vi "Measurement Logic.vi"() -> ()   [LabVIEW 2024, in "NIScopeFrequencyDomain.lvlib"]
uses:
  NIScopeFrequencyDomain.lvlib
  Measurement Configuration.ctl
  Measurement Results.ctl
  <vilib>/gRPC/Generated APIs/ni/protobuf/types/RPC Messages/ni_protobuf_types_DoubleXYData.ctl
  <vilib>/MeasurementLink/MeasurementLink Measurement Server/Measure Call Context/Measure Call Context.lvclass
  <vilib>/MeasurementLink/MeasurementLink Measurement Server/Measure Call Context/Reserve Sessions - 1Pin.vi
  <vilib>/MeasurementLink/MeasurementLink niScope/Initialize Sessions - 1Sess.vi
  <vilib>/MeasurementLink/MeasurementLink niScope/Get Connections - 1Pin 1Conn.vi
  <instrlib>/niScope/Configure/Trigger/niScope Configure Trigger Edge.vi
  <instrlib>/niScope/Acquire/Fetch/niScope Fetch WDT.vi
  <vilib>/MeasurementLink/MeasurementLink niScope/MeasurementLink niScope.lvlib
  <vilib>/gRPC/Generated APIs/ni/protobuf/types/ni.protobuf.types.lvlib
  <vilib>/MeasurementLink/MeasurementLink Session Management V1/Session Reservation/Session Reservation.lvclass
panel:
  out "measure call context out":refnum<class "Measure Call Context.lvclass">
  in  "measure call context in":refnum<class "Measure Call Context.lvclass">
  out "measurement results":T1
  in  "measurement configuration":T3={"Pin Name"="", "Vertical Range (V)"=10.0, "Vertical Offset (V)"=0.0, "Vertical Coupling"=1, "Minimum Sample Rate (S/s)"=10000.0, "Minimum Record Length (S)"=20000, "Trigger Level (V)"=0.0, "Trigger Coupling"=1, "Trigger Slope"=0} {"Trigger Slope" items=["Positive", "Negative"]; "Trigger Coupling" items=["AC"=0, "DC"=1, "HF Reject"=3, "LF Reject"=4, "AC Plus HF Reject"=1001]; "Trigger Level (V)" format="%.2g"; "Minimum Sample Rate (S/s)" format="%#.5p"; "Vertical Coupling" items=["AC", "DC", "Ground"]; "Vertical Offset (V)" format="%.2p"; "Vertical Range (V)" format="%.2f"}
  out "error out":errorcluster
  in  "error in":errorcluster
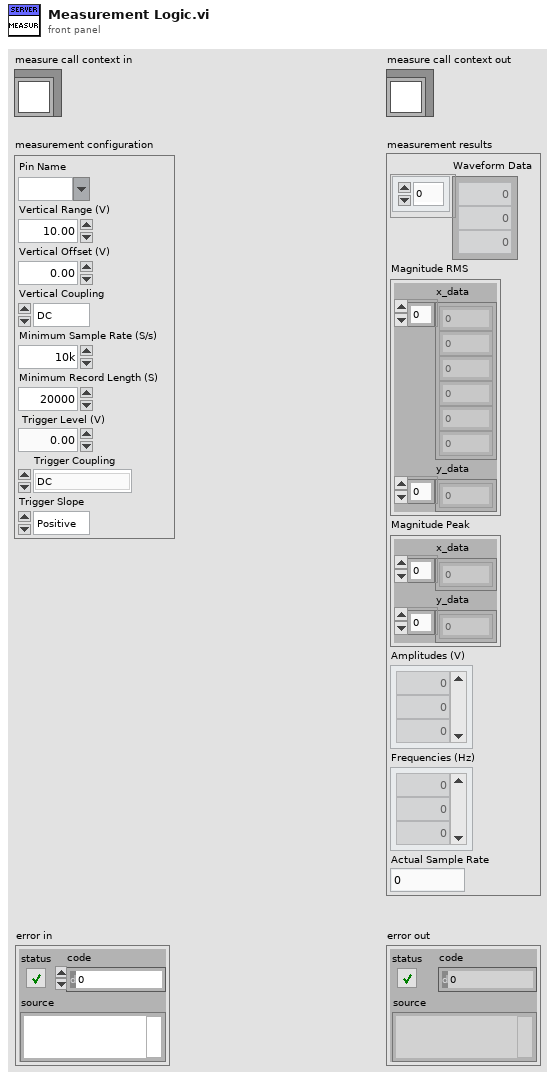
[diagram p1: front panel]
types:
  T1 = typedef "NIScopeFrequencyDomain.lvlib/Measurement Results.ctl" = cluster{"Waveform Data":dbl[], "Magnitude RMS":T2, "Magnitude Peak":T2, "Amplitudes (V)":dbl[], "Frequencies (Hz)":dbl[], "Actual Sample Rate":dbl}
  T2 = typedef "ni.protobuf.types.lvlib/ni_protobuf_types_DoubleXYData.ctl" = cluster{"x_data":dbl[], "y_data":dbl[]}
  T3 = typedef "NIScopeFrequencyDomain.lvlib/Measurement Configuration.ctl" = cluster{"Pin Name":string, "Vertical Range (V)":dbl, "Vertical Offset (V)":dbl, "Vertical Coupling":i32, "Minimum Sample Rate (S/s)":dbl, "Minimum Record Length (S)":i32, "Trigger Level (V)":dbl, "Trigger Coupling":u32, "Trigger Slope":i32}
  T4 = typedef "MeasurementLink niScope.lvlib/Connection with Session.ctl" = cluster{"connection":T5, "session":refnum<k15>}
  T5 = typedef "MeasurementLink Session Management V1.lvlib/Session Reservation.lvclass/Connection.ctl" = cluster{"pin or relay name":string, "site":i32, "instrument type id":string, "channel":string}
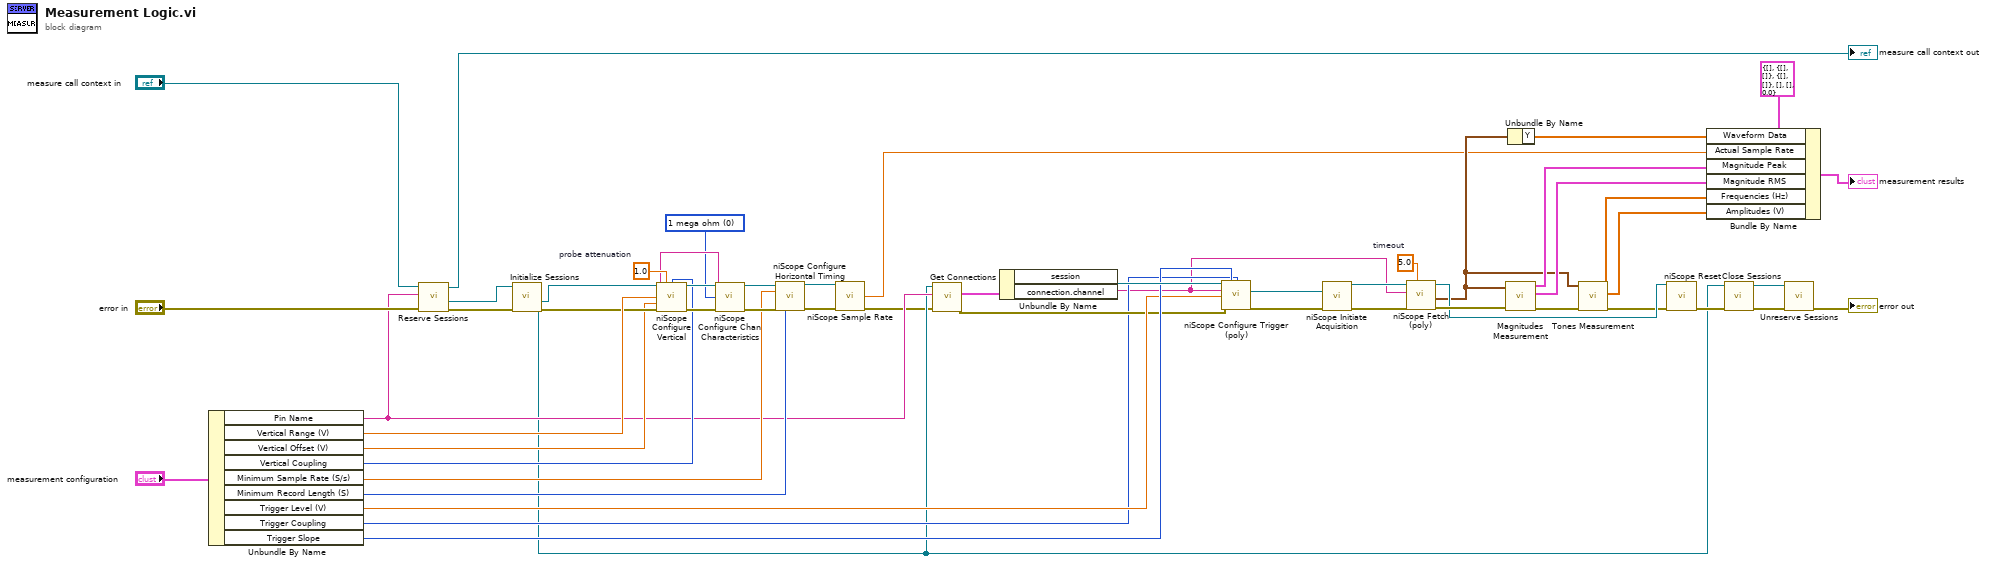
[diagram p0: block diagram]
diagram:
  w13 = u32 0 items=["1 mega ohm"=0, "50 ohms"=2] ("input impedance")
  w24 = 5.0  # timeout
  w44 = 1.0  # probe attenuation
  n1 = Unbundle By Name("measurement configuration") -> ("Pin Name"=w35:string, "Vertical Range (V)"=w47:dbl, "Vertical Offset (V)"=w45:dbl, "Vertical Coupling"=w36:i32, "Minimum Sample Rate (S/s)"=w38:dbl, "Minimum Record Length (S)"=w37:i32, "Trigger Level (V)"=w31:dbl, "Trigger Coupling"=w29:u32, "Trigger Slope"=w32:i32)
  n2 = call-poly <vilib>:"Reserve Sessions.vi"("error in"="error in", "pin or relay name"=w35, "measurement context in"="measure call context in") -> ("error out"=w49:errorcluster, "session reservation out"=w51:refnum<class "Session Reservation.lvclass">, "measurement context out"=→"measure call context out":refnum<class "Measure Call Context.lvclass">)  [unwired: 6 in]
  n3 = call-poly <vilib>:"Initialize Sessions.vi"("error in"=w49, "session reservation in"=w51) -> ("error out"=w46:errorcluster, "channel list"=w41:string, "session"=w48:refnum<k15>, "session reservation out"=w17:refnum<class "Session Reservation.lvclass">)  [unwired: 6 in]
  n4 = call <instrlib>:"niScope Configure Vertical.vi"("instrument handle"=w48, "probe attenuation"=w44, "vertical coupling"=w36, "channels"=w41, "vertical range"=w47, "vertical offset"=w45, "error in"=w46) -> ("instrument handle out"=w43:refnum<k15>, "error out"=w42:errorcluster)  [unwired: 7 in]
  n5 = call <instrlib>:"niScope Configure Chan Characteristics.vi"("instrument handle"=w43, "channels"=w41, "input impedance"=w13, "error in"=w42) -> ("instrument handle out"=w40:refnum<k15>, "error out"=w39:errorcluster)  [unwired: 10 in]
  n6 = call <instrlib>:"niScope Configure Horizontal Timing.vi"("instrument handle"=w40, "min sample rate"=w38, "error in"=w39, "min record length"=w37) -> ("instrument handle out"=w5:refnum<k15>, "error out"=w4:errorcluster)  [unwired: 10 in]
  n7 = call <instrlib>:"niScope Sample Rate.vi"("instrument handle"=w5, "error in"=w4) -> ("actual sample rate"=w1:dbl, "error out"=w3:errorcluster)  [unwired: 11 in, 1 out]
  n8 = call-poly <vilib>:"Get Connections.vi"("error in"=w3, "pin or relay name"=w35, "session reservation in"=w17) -> ("error out"=w30:errorcluster, "connection"=w34:T4)  [unwired: 6 in, 1 out]
  n9 = Unbundle By Name(w34) -> ("session"=w33:refnum<k15>, "connection.channel"=w23:string)
  n10 = call-poly <instrlib>:"niScope Configure Trigger (poly).vi"("instrument handle"=w33, "trigger slope"=w32, "trigger coupling"=w29, "trigger source"=w23, "trigger level"=w31, "error in"=w30) -> ("instrument handle out"=w28:refnum<k15>, "error out"=w27:errorcluster)  [unwired: 8 in]
  n11 = call <instrlib>:"niScope Initiate Acquisition.vi"("instrument handle"=w28, "error in"=w27) -> ("instrument handle out"=w26:refnum<k15>, "error out"=w25:errorcluster)  [unwired: 12 in]
  n12 = call-poly <instrlib>:"niScope Fetch (poly).vi"("timeout"=w24, "error in"=w25, "channels"=w23, "instrument handle"=w26) -> ("error out"=w20:errorcluster, "wfm"=w10:waveform(dbl), "instrument handle out"=w19:refnum<k15>)  [unwired: 4 in, 1 out]
  n13 = call "Magnitudes Measurement.vi"("error in"=w20, "wfm"=w10) -> ("error out"=w9:errorcluster, "Magnitude RMS"=w11:cluster{dbl[], "magnitude":dbl[]}, "Magnitude Peak"=w12:cluster{dbl[], dbl[]})  [unwired: 7 in]
  n14 = Unbundle By Name(w10) -> ("Y"=w2:dbl[])
  n15 = call "Tones Measurement.vi"("error in"=w9, "wfm"=w10) -> ("error out"=w8:errorcluster, "Detected Amplitudes"=w6:dbl[], "Detected Frequencies"=w7:dbl[])  [unwired: 7 in]
  n16 = call <instrlib>:"niScope Reset.vi"("instrument handle"=w19, "error in"=w8) -> ("error out"=w18:errorcluster)  [unwired: 12 in, 1 out]
  n17 = Bundle By Name(cluster=T1 {"Waveform Data"=[], "Magnitude RMS"={"x_data"=[], "y_data"=[]}, "Magnitude Peak"={"x_data"=[], "y_data"=[]}, "Amplitudes (V)"=[], "Frequencies (Hz)"=[], "Actual Sample Rate"=0.0} ("measurement results"), "Waveform Data"=w2, "Actual Sample Rate"=w1, "Magnitude Peak"=w12, "Magnitude RMS"=w11, "Frequencies (Hz)"=w7, "Amplitudes (V)"=w6) -> (→"measurement results":T1)
  n18 = call <vilib>:"Close Sessions.vi"("error in"=w18, "session reservation in"=w17) -> ("error out"=w15:errorcluster, "session reservation out"=w16:refnum<class "Session Reservation.lvclass">)  [unwired: 8 in]
  n19 = call <vilib>:"Unreserve Sessions.vi"("error in"=w15, "session reservation in"=w16) -> ("error out"=→"error out":errorcluster)  [unwired: 9 in]
